vi "WriteDAQ.vi"(7 "Cycle":i32, 8 "error in (no error)":errorcluster, 9 "DigitalWaveform_In":digitalwaveform[](array[waveform]), 10 "AnalogWaveform_In":waveform(dbl)[](array[waveform]), 11 "SetupInfo_IN":T1={"ConfigParameters_Analog"={"JAI camera fps"=240.0, "Bi-Lateral Galvo xy scan range (V)"=0.7, "Bi-Lateral Galvo xy scan frequency (Hz)"=500, "AOM Blind percent (%)"=0.1, "AOM start blind percent (%) "=70.0, "ROI threshold"=1.0, "AO Sampling rate"=1000000.0}, "ConfigParameters_Digital"={"Steps per volume"=25.0, "Time per volume (s)"=0.4, "OG start layer"=15.0, "Objective Lin Rising Vel (micron/ms）"=1.0, "Image depth (micron)"=200.0, "OG latency (s)"=10.0, "OG repitation"=3.0, "OG end layer"=17.0, "Shock1 duration (s)"=0.001, "Shock2 duration (s)"=0.001, "Shock3 duration (s)"=0.01, "Shock4 duration (s)"=0.01, "Shock5 duration (s)"=0.1, "Shock duration_New"=[]}, "ConfigParameters_Other1"={"Frontal Galvo xy scan range (V)"=0.14, "Frontal Galvo xy scan frequency (Hz)"=500, "PFI 0 digital clock frequency"=500000.0, "Window size for layer index"=0.5, "sCMOS fps"=95.0}, "ConfigParameters_Others2"={"#Trials baseline"=6, "#Trials test"=6, "Time before acq. (s)"=360.0, "Time before test (s)"=600.0, "#Blocks acquisition"=5, "Inter-trial interval baseline (s)"=60.0, "#Trials per acquition block"=6, "Inter-block interval acquisition (s)"=360.0, "Inter-trial interval acquisition (s)"=20.0, "Flash latency (s)"=10.0, "Flash duration (s)"=3.2, "Response duration (s)"=10.0, "MaxTimeEventDetection (s)"=6, "StimType"=enum."Flash", "#MaxEvents"=6}, "ProcessParametersOut"={"stand Z vol Acquisition time (s)"=0.2631578947368421, "stand Z vol Backward time (s)"=0.13684210526315793, "Objective scan volt"=5.0, "Bi-lateral Galvo Z scan volt"=0.1800000180000018, "Frontal Galvo Z scan volt"=0.14940000509752818, "Objective step length (micron)"=8.0, "OG Z volet Linear Dec time (s)"=0.024, "OG Z vol Stim. steps time (s)"=0.031578947368421054, "OG Z vol Linear Acc time (s)"=0.112, "#Vol. of flash"=8, "#Vol. of shock"=1, "#Vol. bef flash"=25, "#Vol. aft flash"=17, "OG Z vol Linear Dec time (s)"=0.112, "OG Z vol time (s)"=0.39073684210526316, "Stack duration"=[0.001, 0.001, 0.01, 0.01, 0.1], "AOM stand. value size"=400000, "Plane indexing length"=0, "#Vol. blank"=0, "#Vol. blank before acq"=0, "#Vol. blank before test"=0, " #Inter-block interval acquisition (Ed-St Vol)"=0}, "WaveformParameters"={"stand Z vol Acquisition samp info"={"Fs"=1000000.0, "#s"=263158.0}, "stand Z vol Backward samp info"={"Fs"=1000000.0, "#s"=136842.0}, "OG Z vol Linear Acc samp info"={"Fs"=1000000.0, "#s"=112000.0}, "OG Z vol Stim. steps samp info"={"Fs"=1000000.0, "#s"=31579.0}, "OG Z volet Linear Dec samp info"={"Fs"=1000000.0, "#s"=24000.0}, "OG Z vol Linear Dec samp info"={"Fs"=1000000.0, "#s"=112000.0}, "OG Z vol samp info"={"Fs"=1000000.0, "#s"=390737.0}, "stand Z vol backforth samp info"={"Fs"=1000000.0, "#s"=400000.0}}, "AnalogWaveform"={"Bi-lateral Galvo Z stand waveform"={"t0"=timestamp(0 s since 1904-01-01), "dt"=1.0, "Y"=[]}, "Frontal Galvo Z stand waveform"={"t0"=timestamp(0 s since 1904-01-01), "dt"=1.0, "Y"=[]}, "Bi-lateral Galvo XY stand waveform"={"t0"=timestamp(0 s since 1904-01-01), "dt"=1.0, "Y"=[]}, "Frontal Galvo XY stand waveform"={"t0"=timestamp(0 s since 1904-01-01), "dt"=1.0, "Y"=[]}, "sCMOS stand waveform"={"t0"=timestamp(0 s since 1904-01-01), "dt"=1.0, "Y"=[]}, "Detection objective stand waveform"={"t0"=timestamp(0 s since 1904-01-01), "dt"=1.0, "Y"=[]}, "AOM stand waveform"={"t0"=timestamp(0 s since 1904-01-01), "dt"=1.0, "Y"=[]}, "PFI 0 clock stand waveform"={"t0"=timestamp(0 s since 1904-01-01), "dt"=1.0, "Y"=[]}, "Bi-lateral Galvo Z OG waveform"={"t0"=timestamp(0 s since 1904-01-01), "dt"=1.0, "Y"=[]}, "Bi-lateral Galvo XY OG waveform"={"t0"=timestamp(0 s since 1904-01-01), "dt"=1.0, "Y"=[]}, "Frontal Galvo Z OG waveform"={"t0"=timestamp(0 s since 1904-01-01), "dt"=1.0, "Y"=[]}, "Frontal Galvo XY OG waveform"={"t0"=timestamp(0 s since 1904-01-01), "dt"=1.0, "Y"=[]}, "sCMOS OG waveform"={"t0"=timestamp(0 s since 1904-01-01), "dt"=1.0, "Y"=[]}, "Detection objective OG waveform"={"t0"=timestamp(0 s since 1904-01-01), "dt"=1.0, "Y"=[]}, "AOM OG waveform"={"t0"=timestamp(0 s since 1904-01-01), "dt"=1.0, "Y"=[]}, "PFI 0 clock OG wavee"={"t0"=timestamp(0 s since 1904-01-01), "dt"=1.0, "Y"=[]}, "sCMOS blank waveform"={"t0"=timestamp(0 s since 1904-01-01), "dt"=1.0, "Y"=[]}, "All analog OG wave"=[], "All analog stand wave"=[], "All analog blank wave"=[], "BufferWaveform_Analog"=[], "Bi-lateral Galvo Z XY"={"t0"=timestamp(0 s since 1904-01-01), "dt"=1.0, "Y"=[]}, "Frontal Galvo Z XY"={"t0"=timestamp(0 s since 1904-01-01), "dt"=1.0, "Y"=[]}, "sCMOS Trigger XY"={"t0"=timestamp(0 s since 1904-01-01), "dt"=1.0, "Y"=[]}, "Detection objective XY"={"t0"=timestamp(0 s since 1904-01-01), "dt"=1.0, "Y"=[]}, "AOM XY"={"t0"=timestamp(0 s since 1904-01-01), "dt"=1.0, "Y"=[]}, "Analog_XY"=[]}, "DigitalWaveform"={"AllDigitalStandWave"=[], "AllDigialEvokedWave"=[], "AllDigialOGWave"=[], "AllDigitalPairWave_1"=[], "AllDigitalPairWave_2"=[], "AllDigitalPairWave_3"=[], "AllDigitalPairWave_4"=[], "AllDigitalPairWave_5"=[], "Plane Indexing"={"t0"=timestamp(0 s since 1904-01-01), "dt"=0.0, "Y"={"transitions"=[], "data"=[]}, "error"={"status"=FALSE, "code"=37421928, "source"=""}}, "Plane indexing P0.5 OG"={"t0"=timestamp(0 s since 1904-01-01), "dt"=0.0, "Y"={"transitions"=[], "data"=[]}, "error"={"status"=FALSE, "code"=37421928, "source"=""}}, "AllDigitalPairWaves"=[], "BufferWaveform_Digital"=[], "AllDigitalBlankWave"=[], "Digial_XY"=[], "Digital_XY_flash"=[], "Digial_XY DMD"=[]}, "PhysicalResource"={"PhysicalChannels_AI"="", "PhysicalChannels_AO"="", "PhysicalChannels_DO"="", "Task_AnalogOutput"="", "Task_DigitalOutput"="", "Task_AnalogInput"=""}, "ControlsRef"={"Mode_1"=refnum, "EventDetectionMode"=refnum, "Mode_2A"=refnum, "StimulationMode"=refnum, "Mode_2B"=refnum, "ErrorMeg"=refnum}, "test"=""} {"ConfigParameters_Other1"."Frontal Galvo xy scan frequency (Hz)" min=500 max=500; "ConfigParameters_Other1"."Frontal Galvo xy scan range (V)" min=0.0 max=1.5; "ConfigParameters_Analog"."AOM start blind percent (%)" min=10.0 max=90.0; "ConfigParameters_Analog"."AOM Blind percent (%)" min=0.1 max=100.0; "ConfigParameters_Analog"."Bi-Lateral Galvo xy scan frequency (Hz)" min=500 max=500; "ConfigParameters_Analog"."Bi-Lateral Galvo xy scan range (V)" min=0.0 max=1.5}) -> (0 "error out":errorcluster, 1 "Trigger":bool, 3 "SetupInfo_OUT":T1={"ConfigParameters_Analog"={"JAI camera fps"=240.0, "Bi-Lateral Galvo xy scan range (V)"=0.7, "Bi-Lateral Galvo xy scan frequency (Hz)"=500, "AOM Blind percent (%)"=0.1, "AOM start blind percent (%) "=70.0, "ROI threshold"=1.0, "AO Sampling rate"=1000000.0}, "ConfigParameters_Digital"={"Steps per volume"=25.0, "Time per volume (s)"=0.4, "OG start layer"=15.0, "Objective Lin Rising Vel (micron/ms）"=1.0, "Image depth (micron)"=200.0, "OG latency (s)"=10.0, "OG repitation"=3.0, "OG end layer"=17.0, "Shock1 duration (s)"=0.001, "Shock2 duration (s)"=0.001, "Shock3 duration (s)"=0.01, "Shock4 duration (s)"=0.01, "Shock5 duration (s)"=0.1, "Shock duration_New"=[]}, "ConfigParameters_Other1"={"Frontal Galvo xy scan range (V)"=0.14, "Frontal Galvo xy scan frequency (Hz)"=500, "PFI 0 digital clock frequency"=500000.0, "Window size for layer index"=0.5, "sCMOS fps"=95.0}, "ConfigParameters_Others2"={"#Trials baseline"=6, "#Trials test"=6, "Time before acq. (s)"=360.0, "Time before test (s)"=600.0, "#Blocks acquisition"=5, "Inter-trial interval baseline (s)"=60.0, "#Trials per acquition block"=6, "Inter-block interval acquisition (s)"=360.0, "Inter-trial interval acquisition (s)"=20.0, "Flash latency (s)"=10.0, "Flash duration (s)"=3.2, "Response duration (s)"=10.0, "MaxTimeEventDetection (s)"=6, "StimType"=enum."Flash", "#MaxEvents"=6}, "ProcessParametersOut"={"stand Z vol Acquisition time (s)"=0.2631578947368421, "stand Z vol Backward time (s)"=0.13684210526315793, "Objective scan volt"=5.0, "Bi-lateral Galvo Z scan volt"=0.1800000180000018, "Frontal Galvo Z scan volt"=0.14940000509752818, "Objective step length (micron)"=8.0, "OG Z volet Linear Dec time (s)"=0.024, "OG Z vol Stim. steps time (s)"=0.031578947368421054, "OG Z vol Linear Acc time (s)"=0.112, "#Vol. of flash"=8, "#Vol. of shock"=1, "#Vol. bef flash"=25, "#Vol. aft flash"=17, "OG Z vol Linear Dec time (s)"=0.112, "OG Z vol time (s)"=0.39073684210526316, "Stack duration"=[0.001, 0.001, 0.01, 0.01, 0.1], "AOM stand. value size"=400000, "Plane indexing length"=0, "#Vol. blank"=0, "#Vol. blank before acq"=0, "#Vol. blank before test"=0, " #Inter-block interval acquisition (Ed-St Vol)"=0}, "WaveformParameters"={"stand Z vol Acquisition samp info"={"Fs"=1000000.0, "#s"=263158.0}, "stand Z vol Backward samp info"={"Fs"=1000000.0, "#s"=136842.0}, "OG Z vol Linear Acc samp info"={"Fs"=1000000.0, "#s"=112000.0}, "OG Z vol Stim. steps samp info"={"Fs"=1000000.0, "#s"=31579.0}, "OG Z volet Linear Dec samp info"={"Fs"=1000000.0, "#s"=24000.0}, "OG Z vol Linear Dec samp info"={"Fs"=1000000.0, "#s"=112000.0}, "OG Z vol samp info"={"Fs"=1000000.0, "#s"=390737.0}, "stand Z vol backforth samp info"={"Fs"=1000000.0, "#s"=400000.0}}, "AnalogWaveform"={"Bi-lateral Galvo Z stand waveform"={"t0"=timestamp(0 s since 1904-01-01), "dt"=1.0, "Y"=[]}, "Frontal Galvo Z stand waveform"={"t0"=timestamp(0 s since 1904-01-01), "dt"=1.0, "Y"=[]}, "Bi-lateral Galvo XY stand waveform"={"t0"=timestamp(0 s since 1904-01-01), "dt"=1.0, "Y"=[]}, "Frontal Galvo XY stand waveform"={"t0"=timestamp(0 s since 1904-01-01), "dt"=1.0, "Y"=[]}, "sCMOS stand waveform"={"t0"=timestamp(0 s since 1904-01-01), "dt"=1.0, "Y"=[]}, "Detection objective stand waveform"={"t0"=timestamp(0 s since 1904-01-01), "dt"=1.0, "Y"=[]}, "AOM stand waveform"={"t0"=timestamp(0 s since 1904-01-01), "dt"=1.0, "Y"=[]}, "PFI 0 clock stand waveform"={"t0"=timestamp(0 s since 1904-01-01), "dt"=1.0, "Y"=[]}, "Bi-lateral Galvo Z OG waveform"={"t0"=timestamp(0 s since 1904-01-01), "dt"=1.0, "Y"=[]}, "Bi-lateral Galvo XY OG waveform"={"t0"=timestamp(0 s since 1904-01-01), "dt"=1.0, "Y"=[]}, "Frontal Galvo Z OG waveform"={"t0"=timestamp(0 s since 1904-01-01), "dt"=1.0, "Y"=[]}, "Frontal Galvo XY OG waveform"={"t0"=timestamp(0 s since 1904-01-01), "dt"=1.0, "Y"=[]}, "sCMOS OG waveform"={"t0"=timestamp(0 s since 1904-01-01), "dt"=1.0, "Y"=[]}, "Detection objective OG waveform"={"t0"=timestamp(0 s since 1904-01-01), "dt"=1.0, "Y"=[]}, "AOM OG waveform"={"t0"=timestamp(0 s since 1904-01-01), "dt"=1.0, "Y"=[]}, "PFI 0 clock OG wavee"={"t0"=timestamp(0 s since 1904-01-01), "dt"=1.0, "Y"=[]}, "sCMOS blank waveform"={"t0"=timestamp(0 s since 1904-01-01), "dt"=1.0, "Y"=[]}, "All analog OG wave"=[], "All analog stand wave"=[], "All analog blank wave"=[], "BufferWaveform_Analog"=[], "Bi-lateral Galvo Z XY"={"t0"=timestamp(0 s since 1904-01-01), "dt"=1.0, "Y"=[]}, "Frontal Galvo Z XY"={"t0"=timestamp(0 s since 1904-01-01), "dt"=1.0, "Y"=[]}, "sCMOS Trigger XY"={"t0"=timestamp(0 s since 1904-01-01), "dt"=1.0, "Y"=[]}, "Detection objective XY"={"t0"=timestamp(0 s since 1904-01-01), "dt"=1.0, "Y"=[]}, "AOM XY"={"t0"=timestamp(0 s since 1904-01-01), "dt"=1.0, "Y"=[]}, "Analog_XY"=[]}, "DigitalWaveform"={"AllDigitalStandWave"=[], "AllDigialEvokedWave"=[], "AllDigialOGWave"=[], "AllDigitalPairWave_1"=[], "AllDigitalPairWave_2"=[], "AllDigitalPairWave_3"=[], "AllDigitalPairWave_4"=[], "AllDigitalPairWave_5"=[], "Plane Indexing"={"t0"=timestamp(0 s since 1904-01-01), "dt"=0.0, "Y"={"transitions"=[], "data"=[]}, "error"={"status"=FALSE, "code"=37421928, "source"=""}}, "Plane indexing P0.5 OG"={"t0"=timestamp(0 s since 1904-01-01), "dt"=0.0, "Y"={"transitions"=[], "data"=[]}, "error"={"status"=FALSE, "code"=37421928, "source"=""}}, "AllDigitalPairWaves"=[], "BufferWaveform_Digital"=[], "AllDigitalBlankWave"=[], "Digial_XY"=[], "Digital_XY_flash"=[], "Digial_XY DMD"=[]}, "PhysicalResource"={"PhysicalChannels_AI"="", "PhysicalChannels_AO"="", "PhysicalChannels_DO"="", "Task_AnalogOutput"="", "Task_DigitalOutput"="", "Task_AnalogInput"=""}, "ControlsRef"={"Mode_1"=refnum, "EventDetectionMode"=refnum, "Mode_2A"=refnum, "StimulationMode"=refnum, "Mode_2B"=refnum, "ErrorMeg"=refnum}, "test"=""} {"ConfigParameters_Other1"."Frontal Galvo xy scan frequency (Hz)" min=500 max=500; "ConfigParameters_Other1"."Frontal Galvo xy scan range (V)" min=0.0 max=1.5; "ConfigParameters_Analog"."AOM start blind percent (%)" min=10.0 max=90.0; "ConfigParameters_Analog"."AOM Blind percent (%)" min=0.1 max=100.0; "ConfigParameters_Analog"."Bi-Lateral Galvo xy scan frequency (Hz)" min=500 max=500; "ConfigParameters_Analog"."Bi-Lateral Galvo xy scan range (V)" min=0.0 max=1.5})   [LabVIEW 2018]
uses:
  SetupInfo.ctl
  ConfigParameters_Analog.ctl
  ConfigParameters_Digital.ctl
  ConfigParameters_Others1.ctl
  ConfigParameters_Others2.ctl
  ProcessParametersOut.ctl
  WaveformParameters.ctl
  AnalogWaveform.ctl
  DigitalWaveform.ctl
  PhysicalResource.ctl
  ControlsRef.ctl
  <vilib>/DAQmx/write.llb/DAQmx Write (Digital 1D Wfm NChan NSamp).vi
  <vilib>/DAQmx/write.llb/DAQmx Write (Analog 1D Wfm NChan NSamp).vi
  <vilib>/Waveform/DWDTOps.llb/DWDT Uncompress Digital.vi
  <vilib>/DAQmx/miscellaneous.llb/DAQmx Fill In Error Info.vi
  Trigger_Global.vi
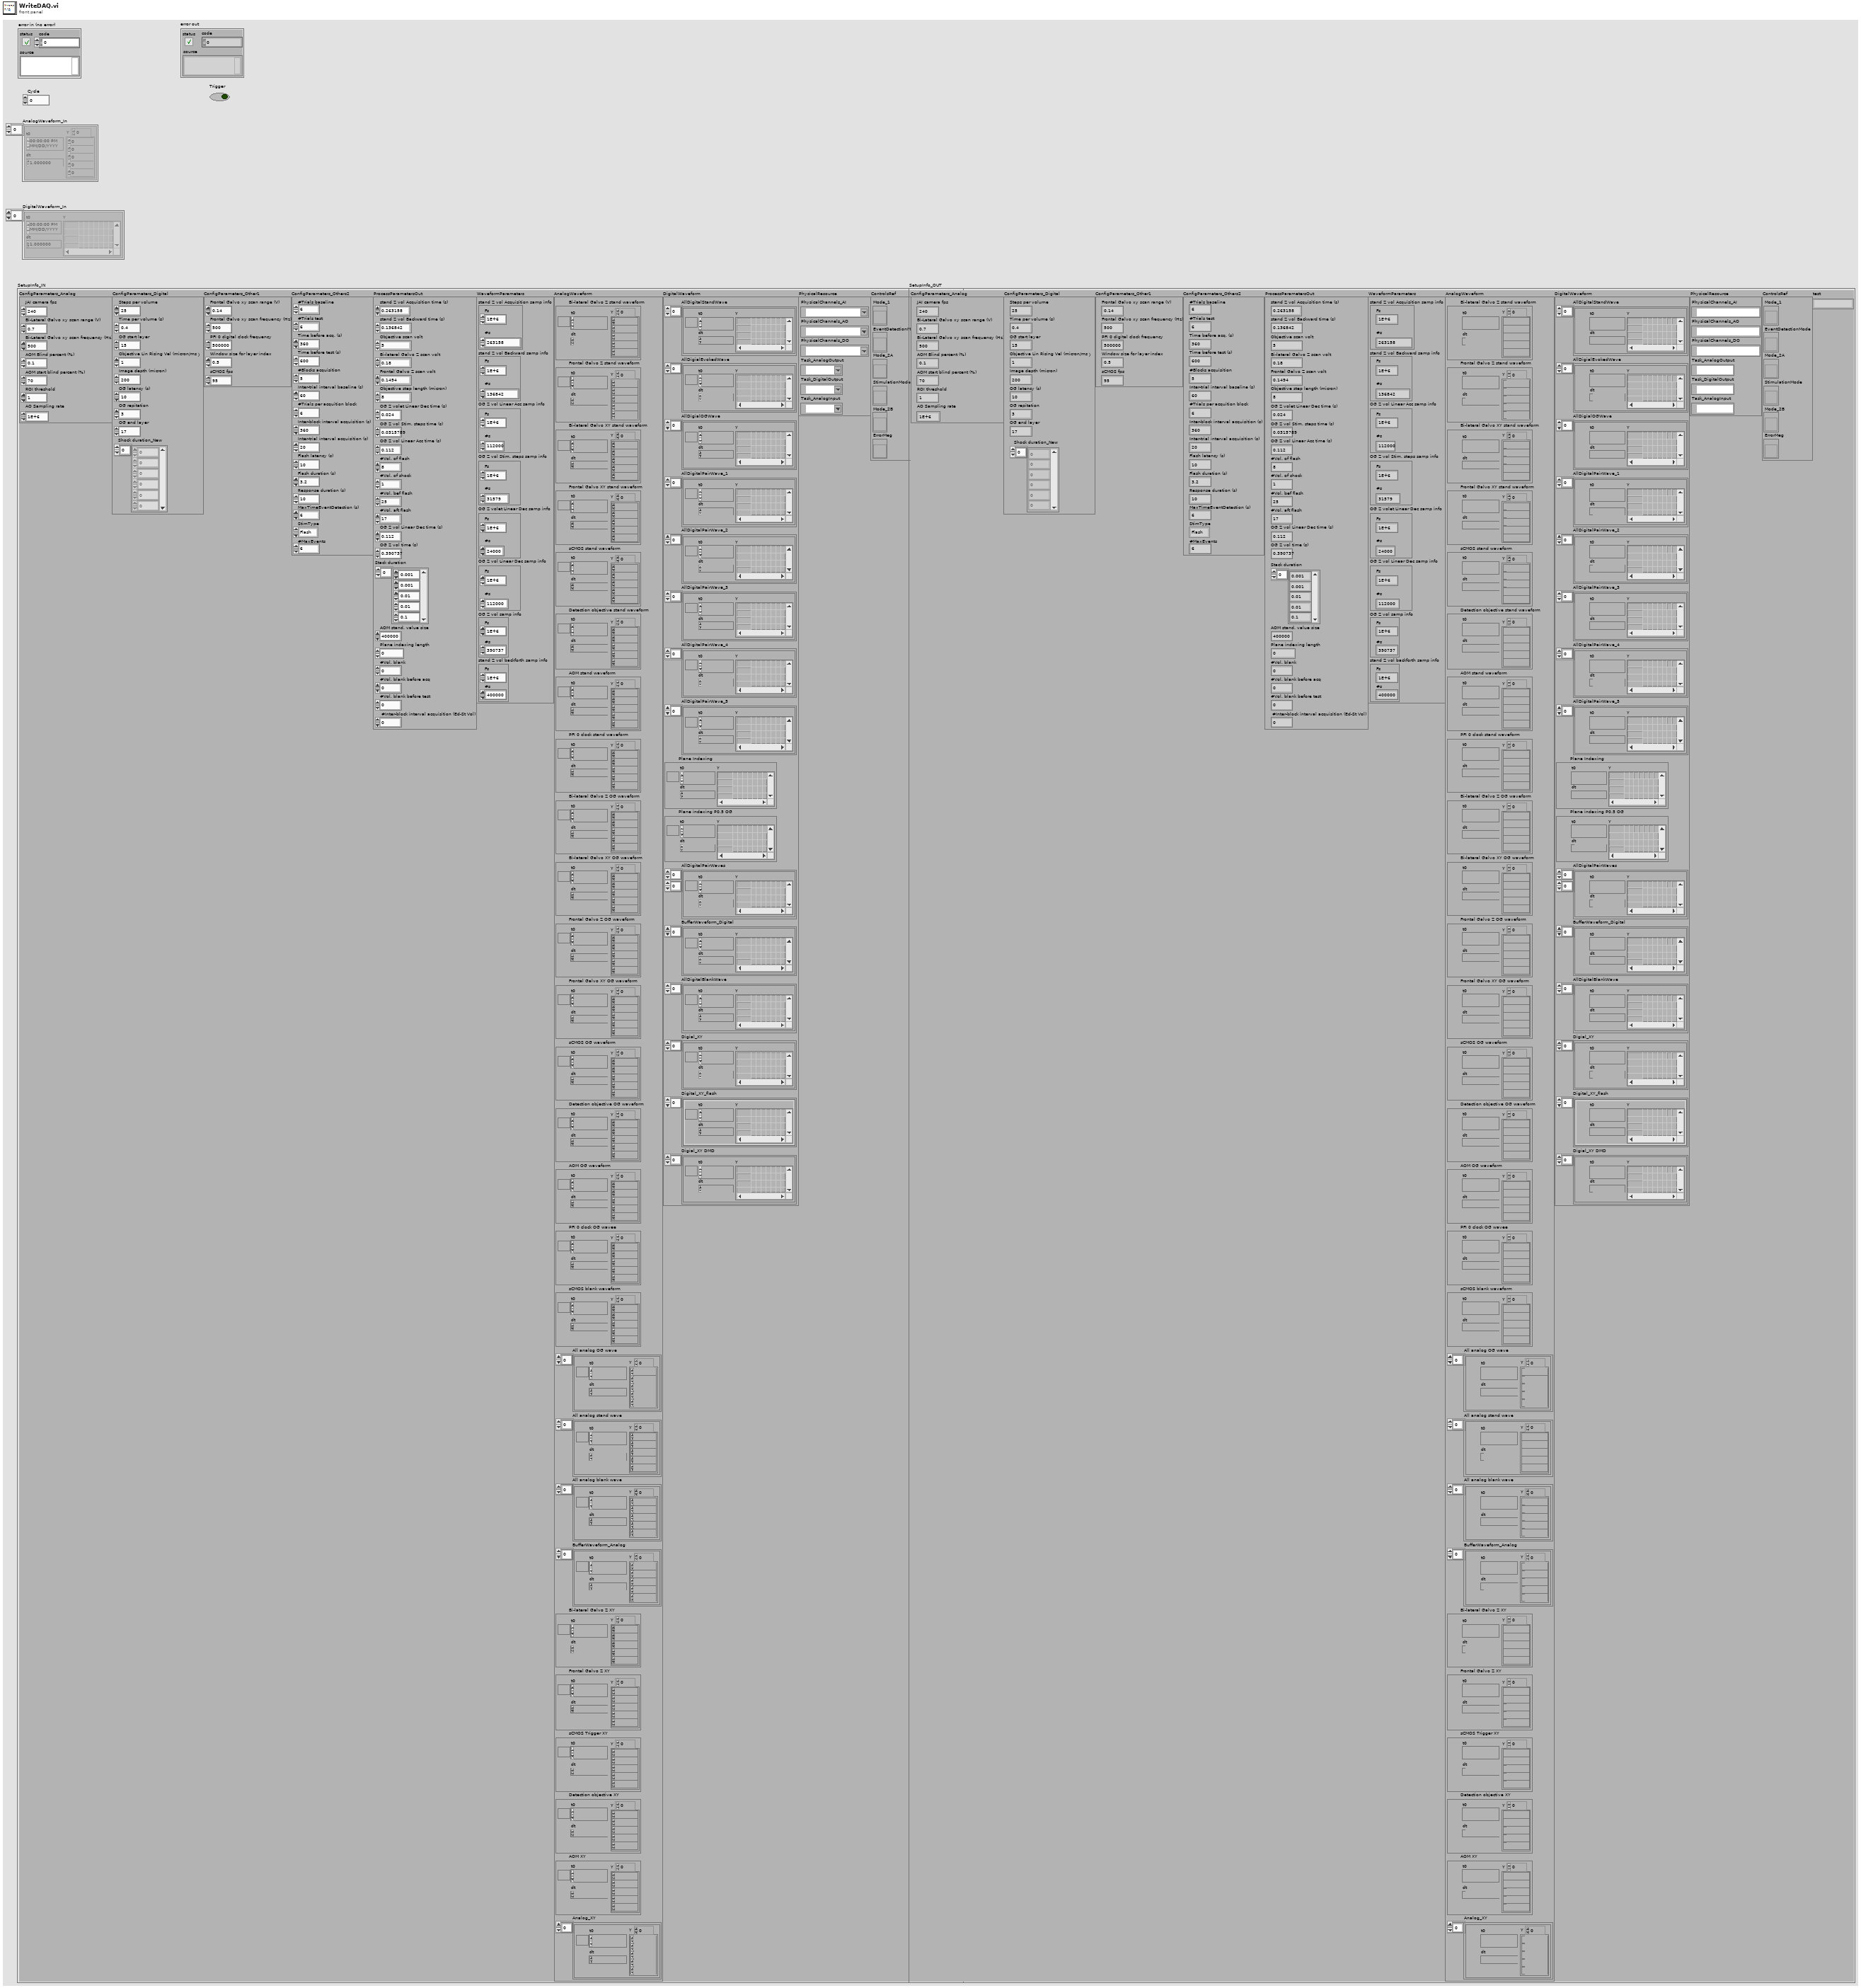
[diagram p1: front panel]
types:
  T1 = typedef "SetupInfo.ctl" = cluster{"ConfigParameters_Analog":T2, "ConfigParameters_Digital":T3, "ConfigParameters_Other1":T4, "ConfigParameters_Others2":T5, "ProcessParametersOut":T6, "WaveformParameters":T7, "AnalogWaveform":T8, "DigitalWaveform":T9, "PhysicalResource":T10, "ControlsRef":T11, "test":string}
  T2 = typedef "ConfigParameters_Analog.ctl" = cluster{"JAI camera fps":dbl, "Bi-Lateral Galvo xy scan range (V)":dbl, "Bi-Lateral Galvo xy scan frequency (Hz)":i16, "AOM Blind percent (%)":dbl, "AOM start blind percent (%) ":dbl, "ROI threshold":dbl, "AO Sampling rate":dbl}
  T3 = typedef "ConfigParameters_Digital.ctl" = cluster{"Steps per volume":dbl, "Time per volume (s)":dbl, "OG start layer":dbl, "Objective Lin Rising Vel (micron/ms）":dbl, "Image depth (micron)":dbl, "OG latency (s)":dbl, "OG repitation":dbl, "OG end layer":dbl, "Shock1 duration (s)":dbl, "Shock2 duration (s)":dbl, "Shock3 duration (s)":dbl, "Shock4 duration (s)":dbl, "Shock5 duration (s)":dbl, "Shock duration_New":dbl[]}
  T4 = typedef "ConfigParameters_Others1.ctl" = cluster{"Frontal Galvo xy scan range (V)":dbl, "Frontal Galvo xy scan frequency (Hz)":i16, "PFI 0 digital clock frequency":dbl, "Window size for layer index":dbl, "sCMOS fps":dbl}
  T5 = typedef "ConfigParameters_Others2.ctl" = cluster{"#Trials baseline":i32, "#Trials test":i32, "Time before acq. (s)":dbl, "Time before test (s)":dbl, "#Blocks acquisition":i32, "Inter-trial interval baseline (s)":dbl, "#Trials per acquition block":i32, "Inter-block interval acquisition (s)":dbl, "Inter-trial interval acquisition (s)":dbl, "Flash latency (s)":dbl, "Flash duration (s)":dbl, "Response duration (s)":dbl, "MaxTimeEventDetection (s)":i32, "StimType":enum16{"Flash", "OG"}, "#MaxEvents":i32}
  T6 = typedef "ProcessParametersOut.ctl" = cluster{"stand Z vol Acquisition time (s)":dbl, "stand Z vol Backward time (s)":dbl, "Objective scan volt":dbl, "Bi-lateral Galvo Z scan volt":dbl, "Frontal Galvo Z scan volt":dbl, "Objective step length (micron)":dbl, "OG Z volet Linear Dec time (s)":dbl, "OG Z vol Stim. steps time (s)":dbl, "OG Z vol Linear Acc time (s)":dbl, "#Vol. of flash":i32, "#Vol. of shock":i32, "#Vol. bef flash":i32, "#Vol. aft flash":i32, "OG Z vol Linear Dec time (s)":dbl, "OG Z vol time (s)":dbl, "Stack duration":dbl[], "AOM stand. value size":i32, "Plane indexing length":i32, "#Vol. blank":i32, "#Vol. blank before acq":i32, "#Vol. blank before test":i32, " #Inter-block interval acquisition (Ed-St Vol)":i32}
  T7 = typedef "WaveformParameters.ctl" = cluster{"stand Z vol Acquisition samp info":cluster{"Fs":dbl, "#s":dbl}, "stand Z vol Backward samp info":cluster{"Fs":dbl, "#s":dbl}, "OG Z vol Linear Acc samp info":cluster{"Fs":dbl, "#s":dbl}, "OG Z vol Stim. steps samp info":cluster{"Fs":dbl, "#s":dbl}, "OG Z volet Linear Dec samp info":cluster{"Fs":dbl, "#s":dbl}, "OG Z vol Linear Dec samp info":cluster{"Fs":dbl, "#s":dbl}, "OG Z vol samp info":cluster{"Fs":dbl, "#s":dbl}, "stand Z vol backforth samp info":cluster{"Fs":dbl, "#s":dbl}}
  T8 = typedef "AnalogWaveform.ctl" = cluster{"Bi-lateral Galvo Z stand waveform":waveform(dbl), "Frontal Galvo Z stand waveform":waveform(dbl), "Bi-lateral Galvo XY stand waveform":waveform(dbl), "Frontal Galvo XY stand waveform":waveform(dbl), "sCMOS stand waveform":waveform(dbl), "Detection objective stand waveform":waveform(dbl), "AOM stand waveform":waveform(dbl), "PFI 0 clock stand waveform":waveform(dbl), "Bi-lateral Galvo Z OG waveform":waveform(dbl), "Bi-lateral Galvo XY OG waveform":waveform(dbl), "Frontal Galvo Z OG waveform":waveform(dbl), "Frontal Galvo XY OG waveform":waveform(dbl), "sCMOS OG waveform":waveform(dbl), "Detection objective OG waveform":waveform(dbl), "AOM OG waveform":waveform(dbl), "PFI 0 clock OG wavee":waveform(dbl), "sCMOS blank waveform":waveform(dbl), "All analog OG wave":waveform(dbl)[], "All analog stand wave":waveform(dbl)[], "All analog blank wave":waveform(dbl)[], "BufferWaveform_Analog":waveform(dbl)[], "Bi-lateral Galvo Z XY":waveform(dbl), "Frontal Galvo Z XY":waveform(dbl), "sCMOS Trigger XY":waveform(dbl), "Detection objective XY":waveform(dbl), "AOM XY":waveform(dbl), "Analog_XY":waveform(dbl)[]}
  T9 = typedef "DigitalWaveform.ctl" = cluster{"AllDigitalStandWave":digitalwaveform[], "AllDigialEvokedWave":digitalwaveform[], "AllDigialOGWave":digitalwaveform[], "AllDigitalPairWave_1":digitalwaveform[], "AllDigitalPairWave_2":digitalwaveform[], "AllDigitalPairWave_3":digitalwaveform[], "AllDigitalPairWave_4":digitalwaveform[], "AllDigitalPairWave_5":digitalwaveform[], "Plane Indexing":digitalwaveform, "Plane indexing P0.5 OG":digitalwaveform, "AllDigitalPairWaves":digitalwaveform[][], "BufferWaveform_Digital":digitalwaveform[], "AllDigitalBlankWave":digitalwaveform[], "Digial_XY":digitalwaveform[], "Digital_XY_flash":digitalwaveform[], "Digial_XY DMD":digitalwaveform[]}
  T10 = typedef "PhysicalResource.ctl" = cluster{"PhysicalChannels_AI":tag, "PhysicalChannels_AO":tag, "PhysicalChannels_DO":tag, "Task_AnalogOutput":refnum<k21>, "Task_DigitalOutput":refnum<k21>, "Task_AnalogInput":refnum<k21>}
  T11 = typedef "ControlsRef.ctl" = cluster{"Mode_1":refnum<vi>, "EventDetectionMode":refnum<vi>, "Mode_2A":refnum<vi>, "StimulationMode":refnum<vi>, "Mode_2B":refnum<vi>, "ErrorMeg":refnum<vi>}
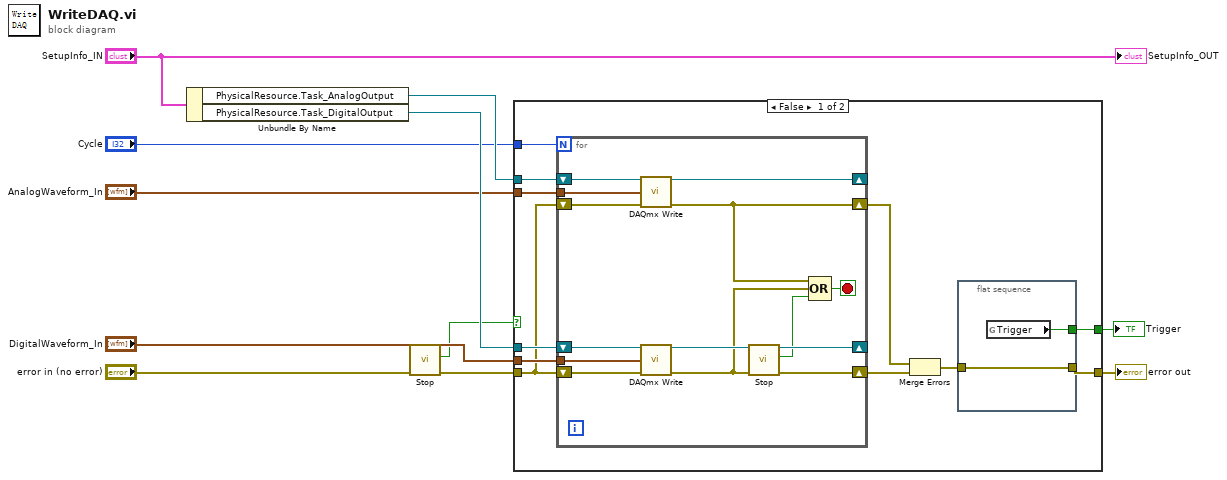
[diagram p0: block diagram]
diagram:
  n1 = Unbundle By Name("SetupInfo_IN") -> ("PhysicalResource.Task_AnalogOutput"=w10:refnum<k21>, "PhysicalResource.Task_DigitalOutput"=w9:refnum<k21>)
  n2 = call "Stop.vi"("error in (no error)"="error in (no error)") -> ("error out"=w3:errorcluster, "StateOut"=w2:bool)  [unwired: 9 in]
  n3 = case shown="False" w2 {
    tunnel: w10 -> [w22 _]
    tunnel: w9 -> [w21 _]
    tunnel: [w13 w38] -> w8
    tunnel: "Cycle" -> [w18 _]
    tunnel: "AnalogWaveform_In" -> [w17 _]
    tunnel: "DigitalWaveform_In" -> [w16 _]
    tunnel: w3 -> [w15 w38]
    tunnel: [w12 _] -> w1
    frame False {
      n4 = for {
        N: w18 -> [_]
        shift-right: [w33] -> _
        shift-left: w22 -> [w37]
        shift-right: [w30] -> w19
        shift-left: w15 -> [w36]
        shift-right: [w32] -> _
        shift-left: w21 -> [w35]
        shift-right: [w28] -> w20
        shift-left: w15 -> [w34]
        tunnel: w17 -> [w26]
        tunnel: w16 -> [w25]
        stop <- w31 stop-if-true
        n5 = call-poly <vilib>:"DAQmx Write.vi"("task/channels in"=w37, "data"=w26, "error in"=w36) -> ("task out"=w33:refnum<k21>, "error out"=w30:errorcluster)  [unwired: 10 in, 1 out]
        n6 = call-poly <vilib>:"DAQmx Write.vi"("task/channels in"=w35, "data"=w25, "error in"=w34) -> ("task out"=w32:refnum<k21>, "error out"=w29:errorcluster)  [unwired: 10 in, 1 out]
        n7 = call "Stop.vi"("error in (no error)"=w29) -> ("error out"=w28:errorcluster, "StateOut"=w27:bool)  [unwired: 9 in]
        n8 = Compound Arithmetic op=OR(w30, w29, w27) -> (w31:bool)
      }
      n9 = Merge Errors(w19, w20) -> (w14:errorcluster)
      n10 = flat-sequence {
        tunnel: w14 -> [w24]
        tunnel: [w24] -> w13
        tunnel: [w23] -> w12
        frame #0 {
          n11 = global read "Trigger_Global.vi" "Trigger"() -> (w23:bool)
        }
      }
    }
    frame True {
    }
  }
  "error out" <- w8
  "Trigger" <- w1
  "SetupInfo_OUT" <- "SetupInfo_IN"
